vi "BoundAngleNeg180to180.vi"(1 "angle":dbl) -> (0 "bound angle":dbl)   [LabVIEW 2017]
doc: "BoundAngleNeg 180to180\nHelp by FRC Team 836 - RoboBees\nVI takes angle input and determines whether the output is 0 to 179.9 or -180 to 0 degrees."
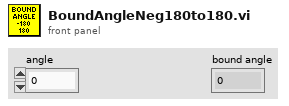
[diagram p1: front panel]
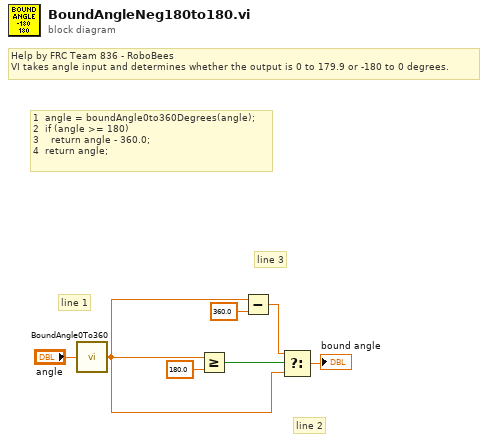
[diagram p0: block diagram]
diagram:
  # "Help by FRC Team 836 - RoboBees\nVI takes angle input and determines whether the output is 0 to 179.9 or -180 to 0 degrees."
  # "line 1"
  # "line 3"
  # "1  angle = boundAngle0to360Degrees(angle);\n2  if (angle >= 180)\n3    return angle - 360.0;\n4  return angle;"
  # "line 2"
  n1 = call <userlib>:"BoundAngle0To360.vi"("angle"="angle") -> ("bound angle"=w2:dbl)
  n2 = Greater Or Equal?(x=w2, y=180.0) -> (x >= y?=w5:bool)
  n3 = Subtract(x=w2, y=360.0) -> (x-y=w4:dbl)
  n4 = Select(t=w4, s=w5, f=w2) -> (s? t:f=→"bound angle":dbl)
